vi "Get SMO Vendor.vi"(8 "error in (no error)":errorcluster, 11 "Inst.FP in":refnum<class "Inst.FP.lvclass">) -> (0 "error out":errorcluster, 2 "SMO Vendor":string, 3 "Inst.FP out":refnum<class "Inst.FP.lvclass">)   [LabVIEW 2019, in "Inst.FP.lvclass"]
doc: "Override this VI to return the vendor or manufacturer of your Instrument"
uses:
  Inst.FP.lvclass
  <userlib>/LevyLab/Instrument Framework/Instrument Types/Cryostat/Instrument.Cryostat.lvclass
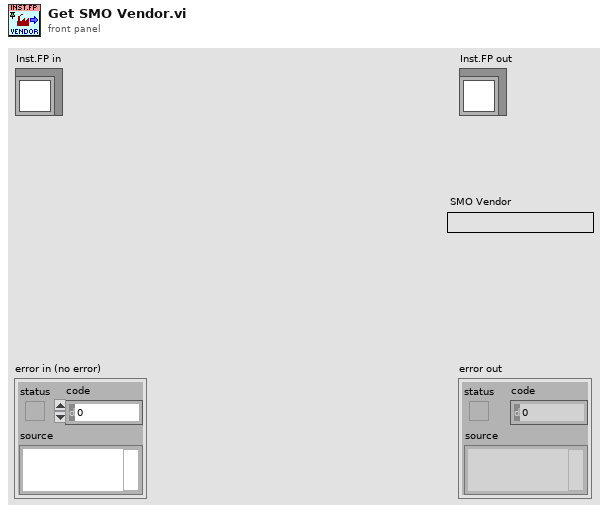
[diagram p1: front panel]
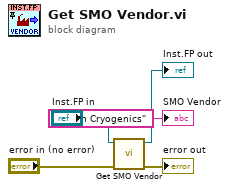
[diagram p0: block diagram]
diagram:
  n1 = call-parent "Get SMO Vendor.vi"("error in (no error)"="error in (no error)", "Instrument in"="Inst.FP in") -> ("error out"=→"error out":errorcluster, "Instrument out"=→"Inst.FP out":refnum<class "Inst.FP.lvclass">)  [unwired: 7 in, 1 out]
  "SMO Vendor" <- "Leiden Cryogenics" ("SMO Vendor")
